vi "Pre Launch Init.vi"(11 "Filled Text Fields Actor in":refnum<class "Filled Text Fields Actor.lvclass">) -> (0 "error out":errorcluster, 3 "Filled Text Fields Actor out":refnum<class "Filled Text Fields Actor.lvclass">)   [LabVIEW 2017, in "Filled Text Fields Actor.lvlib" / "Filled Text Fields Actor.lvclass"]
doc: "(<B>Filename</B>: Actor Framework.lvlib:Actor.lvclass:Pre Launch Init.vi)\n\nDefines behavior that occurs after the Launch Nested Actor method is invoked but before the actor's Actor Core method begins running.\n\nBy default, this method does nothing. A descendant class may override it to define behavior."
uses:
  Filled Text Fields Actor.lvclass
  Filled Text Fields Actor.lvclass/Filled Text Fields Actor.ctl
  <vilib>/ActorFramework/Actor/Actor.lvclass
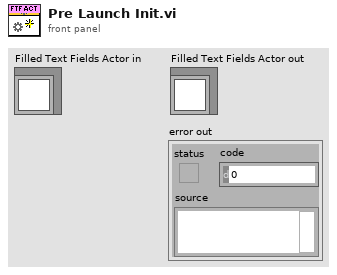
[diagram p1: front panel]
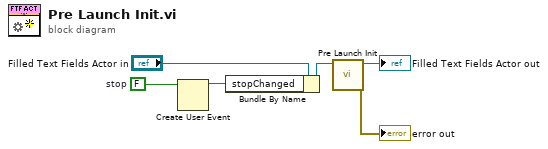
[diagram p0: block diagram]
diagram:
  w3 = FALSE  # stop
  n1 = Create User Event(user event datatype=w3) -> (user event=w1:refnum<user-event>)  [unwired: 1 in, 1 out]
  n2 = Bundle By Name(cluster="Filled Text Fields Actor in", "stopChanged"=w1) -> (w2:refnum<class "Filled Text Fields Actor.lvclass">)
  n3 = call-parent "Pre Launch Init.vi"("Actor in"=w2) -> ("error out"=→"error out":errorcluster, "Actor out"=→"Filled Text Fields Actor out":refnum<class "Filled Text Fields Actor.lvclass">)  [unwired: 9 in]
